vi "NI VeriStand - Close Fault Manager Reference.vi"(8 "error in (no error)":errorcluster, 11 "ChannelFault":T1) -> (0 "error out":errorcluster)   [LabVIEW 2020, in "NI_VS ChannelFault ExecutionAPI.lvlib"]
doc: "Closes an open reference to the channel fault manager on the VeriStand Gateway. Use this VI to close each channel fault manager reference that you open with the Open Fault Manager Reference VI."
uses:
  <vilib>/NI VeriStand/Execution/ChannelFaultManager/NI_VS ChannelFault ExecutionAPI.lvlib
  <vilib>/NI VeriStand/Execution/ChannelFaultManager/ChannelFaultAPI.ctl
  NationalInstruments.VeriStand.ClientAPI
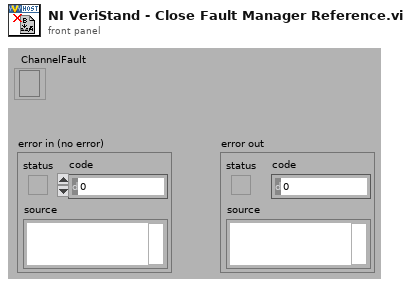
[diagram p1: front panel]
types:
  T1 = typedef "NI_VS ChannelFault ExecutionAPI.lvlib/ChannelFaultAPI.ctl" = refnum<k24>
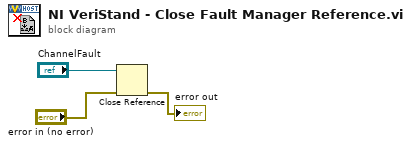
[diagram p0: block diagram]
diagram:
  n1 = Close Reference(reference="ChannelFault", error in (no error)="error in (no error)") -> (error out=→"error out":errorcluster)
